vi "TSCAN_Init.vi"(8 "错误输入（无错误）":errorcluster, 11 "路径输入":path) -> (0 "错误输出":errorcluster, 3 "路径输出":path, 4 "Init_TS_API_Successfully":bool)   [LabVIEW 2019]
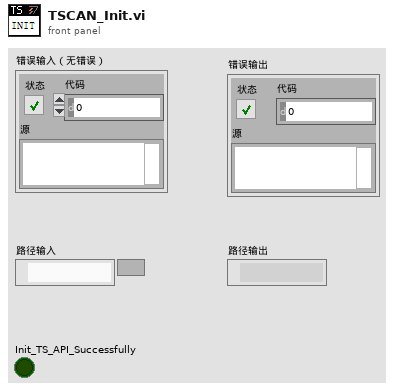
[diagram p1: front panel]
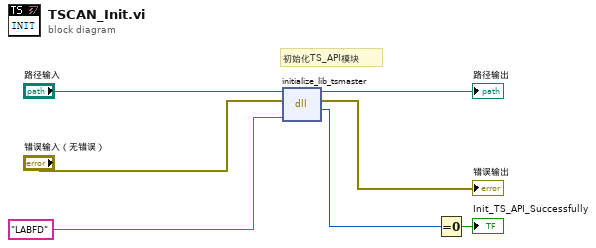
[diagram p0: block diagram]
diagram:
  # "初始化TS_API模块"
  n1 = dll-call lib="PTH2Habs CUsers\nAdministratorDesktopTS_Can通讯PathTSMaster.dll" fn="initialize_lib_tsmaster"(path in="路径输入", error in="错误输入（无错误）", "AppName"="LABFD") -> (path out=→"路径输出":path, error out=→"错误输出":errorcluster, "Initialize_lib_tsmaster"=w6:i32)  [unwired: 2 in]
  n2 = Equal To 0?(x=w6) -> (x = 0?=→"Init_TS_API_Successfully":bool)
